vi "WFS Create Default User Reference.vi"(8 "error in (no error)":errorcluster {"code" format="%.0x"}, 11 "instrument handle":refnum<visa-resource-name>) -> (0 "error out":errorcluster {"code" format="%.0x"}, 3 "instrument handle out":refnum<visa-resource-name>)   [LabVIEW 2020]
doc: "This VI generates a default User Reference which is identical to the Internal Reference. Use VI GetSpotReferencePositions to get the data arrays."
uses:
  WFS_32.dll
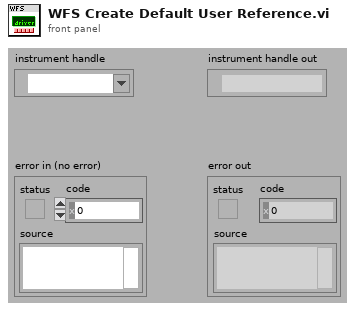
[diagram p1: front panel]
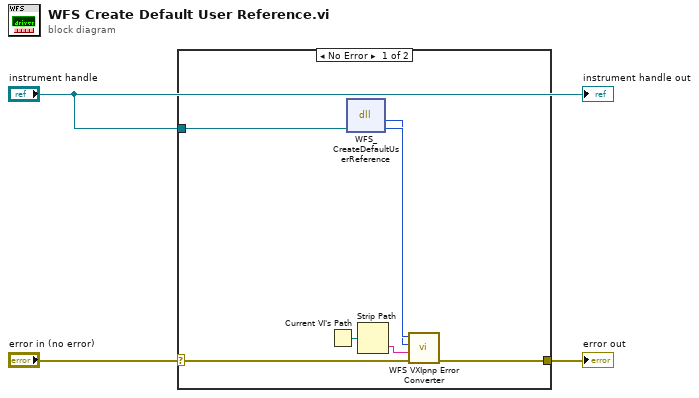
[diagram p0: block diagram]
diagram:
  n1 = case shown="No Error" "error in (no error)" {
    selector: "error in (no error)" -> [w5 w11]
    tunnel: [w4 w11] -> w3
    tunnel: "instrument handle" -> [w9 _]
    frame No Error {
      n2 = Current VI's Path() -> (path=w10:path)
      n3 = dll-call lib="WFS_*.*" fn="WFS_CreateDefaultUserReference"("Instrument Handle"=w9) -> (w7:i32, "Instrument Handle"=w8:u32)  [unwired: 3 in, 2 out]
      n4 = Strip Path(path=w10) -> (name=w6:string)  [unwired: 1 out]
      n5 = call "WFS VXIpnp Error Converter.vi"("error in (no error)"=w5, "Name Of VI (\"\")"=w6, "CVI Error Code (0)"=w7, "instrument handle"=w8) -> ("error out"=w4:errorcluster)  [unwired: 6 in, 1 out]
    }
    frame Error {
    }
  }
  "error out" <- w3
  "instrument handle out" <- "instrument handle"
